vi "z_N[Lambda_0,T,W]_Analytical.vi"(7 "Harmonic f":ext, 8 "N":i32, 9 "W":ext, 10 "T":ext) -> (0 "(T-w)/theta integer":bool, 3 "z_n,N,W(0)":cxt)   [LabVIEW 2019]
panel:
  out "integer r":dbl
  out "r":dbl
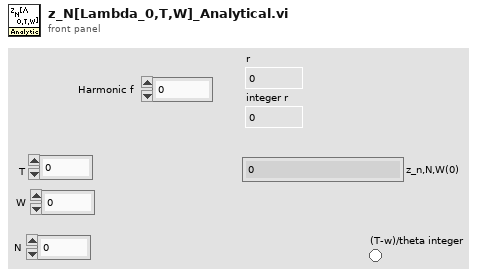
[diagram p1: front panel]
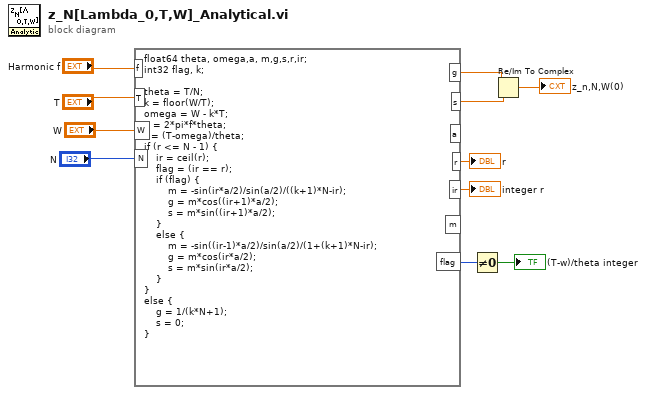
[diagram p0: block diagram]
diagram:
  n1 = formula code="float64 theta, omega,a, m,g,s,r,ir;\nint32 flag, k;\n\ntheta = T/N;\nk = floor(W/T);\nomega = W - k*T;\na = 2*pi*f*theta;\nr = (T-omega)/theta;\nif (r <= N - 1) {\n    ir = ceil(r);\n    flag = (ir == r);\n    if (flag) {\n        m = -sin(ir*a/2)/sin(a/2)/((k+1)*N-ir);\n        g = m*cos((ir+1)*a/2);\n        s = m*sin((ir+1)*a/2);\n    }\n    else {\n        m = -sin((ir-1)*a/2)/sin(a/2)/(1+(k+1)*N-ir);\n        g = m*cos(ir*a/2);\n        s = m*sin(ir*a/2);\n    }\n} \nelse {\n    g = 1/(k*N+1);\n    s = 0;\n}"("f"="Harmonic f", "T"="T", "W"="W", "N"="N") -> ("g"=w7:dbl, "s"=w6:dbl, "r"=→"r":dbl, "flag"=w4:i32, "ir"=→"integer r":dbl)  [unwired: 2 out]
  n2 = Not Equal To 0?(x=w4) -> (x != 0?=→"(T-w)/theta integer":bool)
  n3 = Re/Im To Complex(1:w6, 2:w7) -> (0:→"z_n,N,W(0)":cdb)
